vi "Get Frame Size.vi"(8 "error in (no error)":errorcluster, 9 "nHeight":u16, 10 "nWidth":u16, 11 "nSensorIP":u32) -> (0 "error out":errorcluster, 1 "nHeight out":u16, 2 "nWidth out":u16, 3 "function return":i32)   [LabVIEW 2017, in "imgAcquisiotn.lvlib"]
doc: "DLLFunction int __stdcall ImageCapGetFrameSize(unsigned int nSensorIP, unsigned short* nWidth, unsigned short* nHeight);"
uses:
  imgAcquisiotn.lvlib
  lib/ImageCaptureDLL.dll
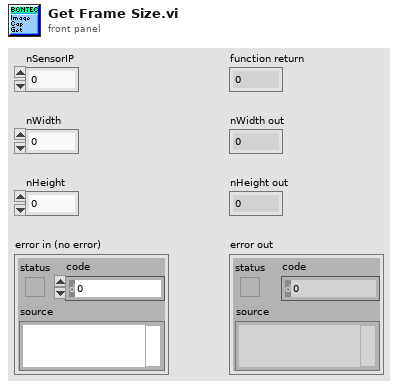
[diagram p1: front panel]
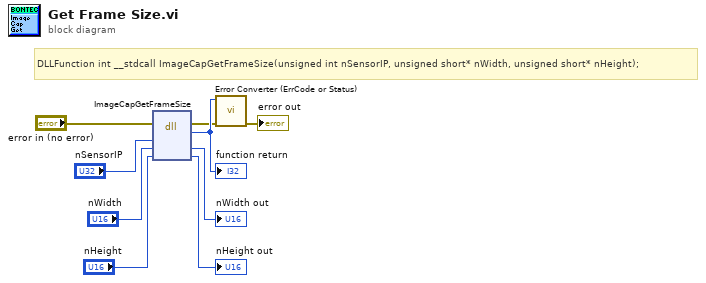
[diagram p0: block diagram]
diagram:
  # "DLLFunction int __stdcall ImageCapGetFrameSize(unsigned int nSensorIP, unsigned short* nWidth, unsigned short* nHeight);"
  n1 = dll-call lib="F:/BonTechFlatPanelLVDriver/lib/ImageCaptureDLL.*" fn="ImageCapGetFrameSize"(error in="error in (no error)", "nSensorIP"="nSensorIP", "nWidth"="nWidth", "nHeight"="nHeight") -> (error out=w2:errorcluster, w9:i32, "nWidth"=→"nWidth out":u16, "nHeight"=→"nHeight out":u16)  [unwired: 3 in, 1 out]
  "function return" <- w9
  n2 = call "Error Converter (ErrCode or Status).vi"("error in (no error)"=w2, "error code"=w9) -> ("error out"=→"error out":errorcluster)  [unwired: 9 in]
